vi "httpProducer.vi"() -> ()   [LabVIEW 2022 SP3]
panel:
  out "Structure":string="{\n\t\"type\": \"sample\" | \"image\" | \"summary\" | \"delete\",\n\t\"data\": {\n      ...\n    }\n}"
  out "delete Data":string="  {\n    \"sampleId\": \"984658168FER4654\"\n  }\n"
  out "summary Data":string="  {\n    \"sampleId\": \"984658168FER4654\",\n    \"maxFeretDiameterMax\": 1568,\n    \"maxFeretDiameterMean\": 1257.5,\n    \"maxFeretDiameterStdDev\": 3.5,\n    \"perimeterMean\": 1456.8,\n    \"perimeterStdDev\": 4.5,\n    \"areaMean\": 12384.4,\n    \"areaStdDev\": 56.4,\n    \"holesMean\": 354.2,\n    \"holesStdDev\": 23.4,\n    \"areaHolesMean\": 12623.2,\n    \"areaHolesStdDev\": 64.3,\n    \"numberOfImages\": 27\n  }\n"
  out "image Data":string="  {\n    \"sampleId\": \"984658168FER4654\",\n    \"speciesName\": \"Spider\",\n    \"date\": \"2022-20-10\",\n    \"imageName\": \"cam1_001\",\n    \"cameraNumber\": 1,\n    \"imageNumber\": 1,\n    \"maxFeretDiameter\": 367,\n    \"perimeter\": 15678,\n    \"area\": 5461,\n    \"holes\": 453,\n    \"areaHoles\": 5914,\n    \"roiLeft\": 0,\n    \"roiTop\": 50,\n    \"roiRight\": 461,\n    \"roiBottom\": 511\n  }\n"
  out "sample Data":string="  \"data\": {\n    \"sampleId\": \"984658168FER4654\",\n    \"projectId\": \"2000146\",\n    \"voucherId\": \"#26413\",\n    \"speciesName\": \"Spider\",\n    \"collectionDate\": \"2022-10-20\",\n    \"sampleStation\": \"Denmark\",\n    \"location\": \"Denmark\",\n    \"lat\": 10.200806,\n    \"lon\": 56.144019,\n    \"determiner\": \"MRJ\",\n    \"sex\": \"Male\",\n    \"exposureTime\": 2000,\n    \"framerate\": 50,\n    \"lightIntensityPct\": 100,\n    \"aperture\": 8,\n    \"operatorName\": \"MRJ\",\n    \"date\": \"2022-20-10\",\n    \"otherNotes\": \"TestPackage\"\n  }"
  in  "RequestToken":bool
  in  "Send":bool
  in  "Stop":bool
  in  "Token":string
  out "Response":string="<!DOCTYPE html>\r\n<html><head><title>Not Found</title></head>\r\n<body>\r\n<h2>Access Error: 404 -- Not Found</h2>\r\n<pre>Cannot open document for: /api/send</pre>\r\n</body>\r\n</html>\r\n"
  in  "Message":string="{\n\t\"type\": \"sample\" ,\n  \"data\": {\n    \"sampleId\": \"984658168FER4654\",\n    \"projectId\": \"2000146\",\n    \"voucherId\": \"#26413\",\n    \"speciesName\": \"Spider\",\n    \"collectionDate\": \"2022-10-20\",\n    \"sampleStation\": \"Denmark\",\n    \"location\": \"Denmark\",\n    \"lat\": 10.200806,\n    \"lon\": 56.144019,\n    \"determiner\": \"MRJ\",\n    \"sex\": \"Male\",\n    \"exposureTime\": 2000,\n    \"framerate\": 50,\n    \"lightIntensityPct\": 100,\n    \"aperture\": 8,\n    \"operatorName\": \"MRJ\",\n    \"date\": \"2022-20-10\",\n    \"otherNotes\": \"TestPackage\"\n  }\n}"
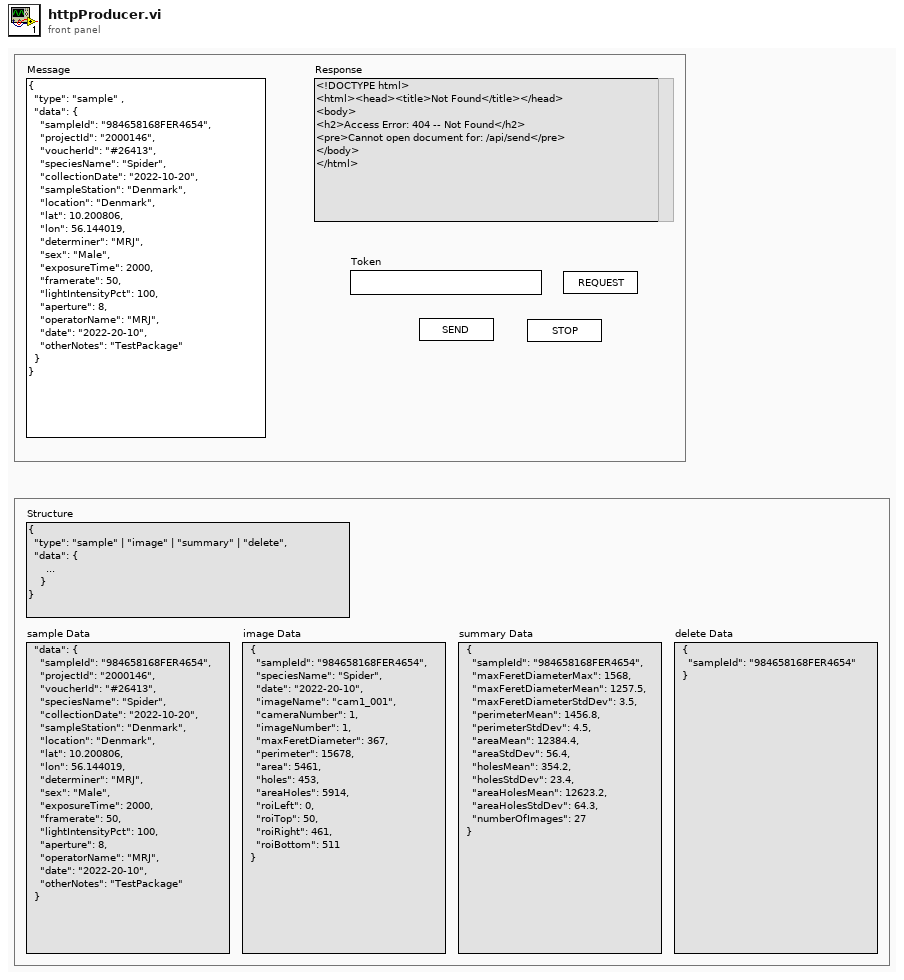
[diagram p1: front panel]
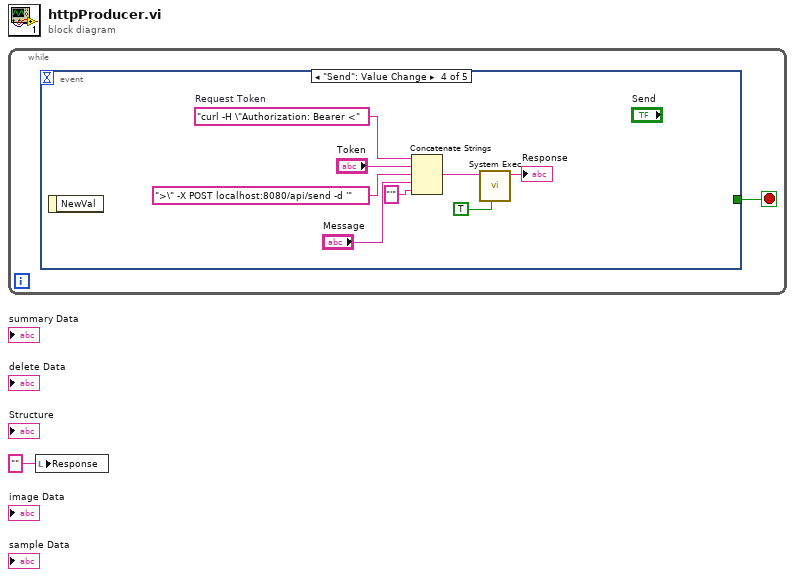
[diagram p0: block diagram]
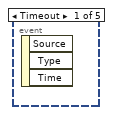
[diagram p2: hidden frame]
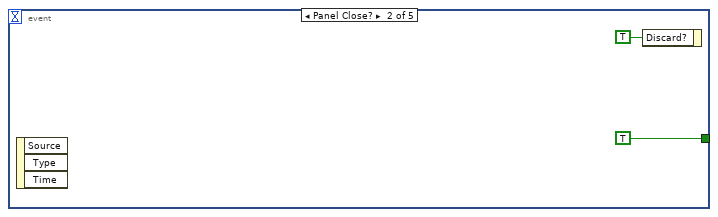
[diagram p3: hidden frame]
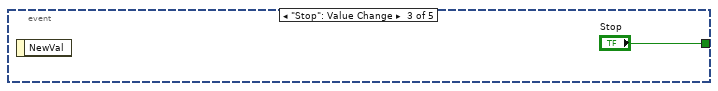
[diagram p4: hidden frame]
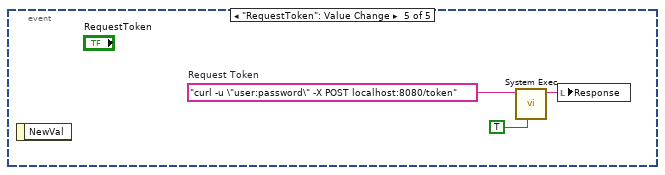
[diagram p5: hidden frame]
diagram:
  n1 = while {
    stop <- w2 stop-if-true
    n2 = event shown="[3] \"Send\": Value Change" {
      selector: _ -> [_ _ _ _ _]
      dyn-events: _ -> [_ _ _ _ _]
      timeout: _ -> [_ _ _ _ _]
      tunnel: [_ TRUE ("Stop") "Stop" _ _] -> w2
      event Timeout {
        n3 = event-data() -> ()  [unwired: 1 in, 3 out]
      }
      event Panel Close? {
        n4 = event-data() -> ()  [unwired: 1 in, 3 out]
        n5 = event-data("Discard?"=TRUE) -> ()  [unwired: 1 in, 1 out]
      }
      event "Stop": Value Change {
        n6 = event-data() -> ()  [unwired: 1 in, 1 out]
      }
      event "Send": Value Change {
        w9 = "curl -H \"Authorization: Bearer <"  # Request Token
        n7 = event-data() -> ()  [unwired: 1 in, 1 out]
        n8 = Concatenate Strings(w9, "Token", ">\" -X POST localhost:8080/api/send -d '" ("string"), "Message", "'" ("string")) -> (w6:string)
        n9 = call <vilib>:"System Exec.vi"("run minimized? (F)"=TRUE, "command line"=w6) -> ("standard output"=→"Response":string)  [unwired: 6 in, 3 out]
      }
      event "RequestToken": Value Change {
        w15 = "curl -u \"user:password\" -X POST localhost:8080/token"  # Request Token
        n10 = event-data() -> ()  [unwired: 1 in, 1 out]
        n11 = call <vilib>:"System Exec.vi"("run minimized? (F)"=TRUE, "command line"=w15) -> ("standard output"=w14:string)  [unwired: 6 in, 3 out]
        n12 = local write "Response"(w14) -> ()
      }
    }
  }
  n13 = local write "Response"("" ("response")) -> ()
